vi "Write Cell.vi"(8 "error in":errorcluster, 10 "Cell":u8, 11 "Change Filter Position MSG in":refnum<class "Change Filter Position MSG.lvclass">) -> (0 "error out":errorcluster, 3 "Change Filter Position MSG out":refnum<class "Change Filter Position MSG.lvclass">)   [LabVIEW 2017, in "Controller.lvlib" / "Change Filter Position MSG.lvclass"]
uses:
  Change Filter Position MSG.lvclass
  Change Filter Position MSG.lvclass/Change Filter Position MSG.ctl
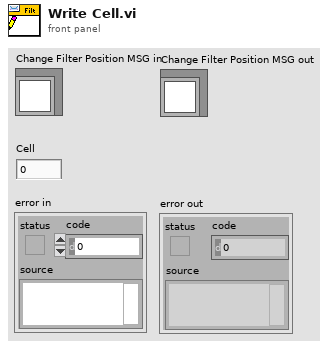
[diagram p1: front panel]
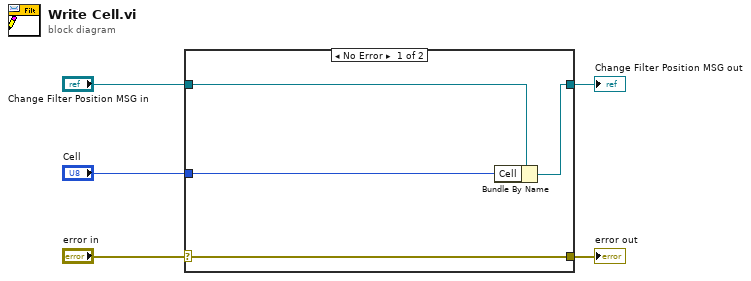
[diagram p0: block diagram]
diagram:
  n1 = case shown="No Error" "error in" {
    selector: "error in" -> [w9 w10]
    tunnel: [w9 w10] -> w4
    tunnel: [w7 w11] -> w2
    tunnel: "Change Filter Position MSG in" -> [w8 w11]
    tunnel: "Cell" -> [w6 _]
    frame No Error {
      n2 = Bundle By Name(cluster=w8, "Cell"=w6) -> (w7:refnum<class "Change Filter Position MSG.lvclass">)
    }
    frame Error {
    }
  }
  "error out" <- w4
  "Change Filter Position MSG out" <- w2
